vi "phasor diagram.vi"() -> ()   [LabVIEW 2017]
panel:
  in  "stop":bool
  out "phasor diagram":cluster{dbl, dbl}[](graph)
  in  "phase angle":dbl
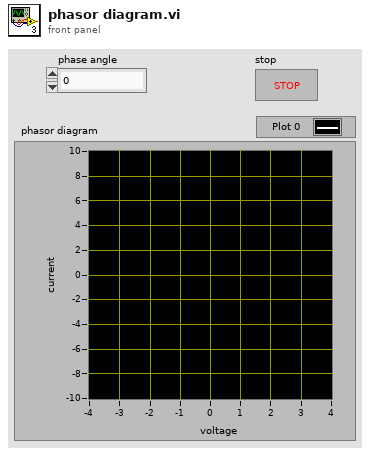
[diagram p1: front panel]
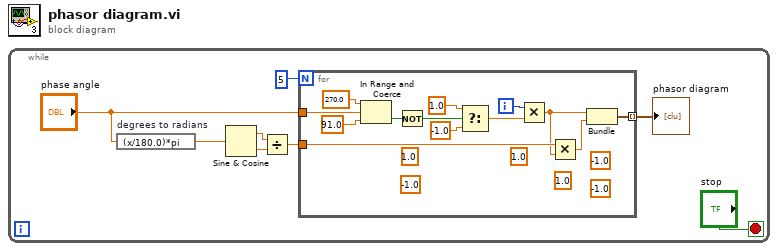
[diagram p0: block diagram]
diagram:
  n1 = while {
    stop <- "stop" stop-if-true
    n2 = expression code="(x/180.0)*pi" "degrees to radians"("phase angle") -> (w8:dbl)
    n3 = Sine & Cosine(0:w8) -> (1:w5:dbl, 2:w4:dbl)
    n4 = Divide(x=w5, y=w4) -> (x/y=w6:dbl)
    n5 = for {
      N: 5 -> [_]
      tunnel: w6 -> [w21]
      tunnel: [w20] -> w7 mode=indexing
      tunnel: "phase angle" -> [w11]
      i -> [w17]
      (unwired) -1.0 ("f")
      (unwired) 1.0 ("t")
      (unwired) -1.0 ("f")
      (unwired) 1.0 ("t")
      (unwired) -1.0 ("f")
      (unwired) 1.0 ("t")
      n6 = In Range and Coerce(upper limit=270.0, x=w11, lower limit=91.0) -> (In Range?=w10:bool)  [unwired: 1 out]
      n7 = Not(x=w10) -> (.not. x?=w9:bool)
      n8 = Select(t=1.0, s=w9, f=-1.0) -> (s? t:f=w16:dbl)
      n9 = Multiply(x=w17, y=w16) -> (x*y=w18:dbl)
      n10 = Multiply(x=w21, y=w18) -> (x*y=w19:dbl)
      n11 = Bundle(w18, w19) -> (w20:cluster{dbl, dbl})  [unwired: 1 in]
    }
    "phasor diagram" <- w7
  }
